vi "作业4和5 .vi"() -> ()   [LabVIEW 2018]
panel:
  in  "输入":dbl
  out "累加值":dbl
  out "等级":string
  in  "成绩":dbl
  out "是否是素数":bool
  in  "input":dbl
  out "求和":dbl
  out "布尔5":bool
  out "布尔4":bool
  out "布尔3":bool
  out "布尔2":bool
  out "布尔1":bool
  in  "间隔时间（ms）":dbl(slide) scale=0.0..1000.0
  in  "停止":bool
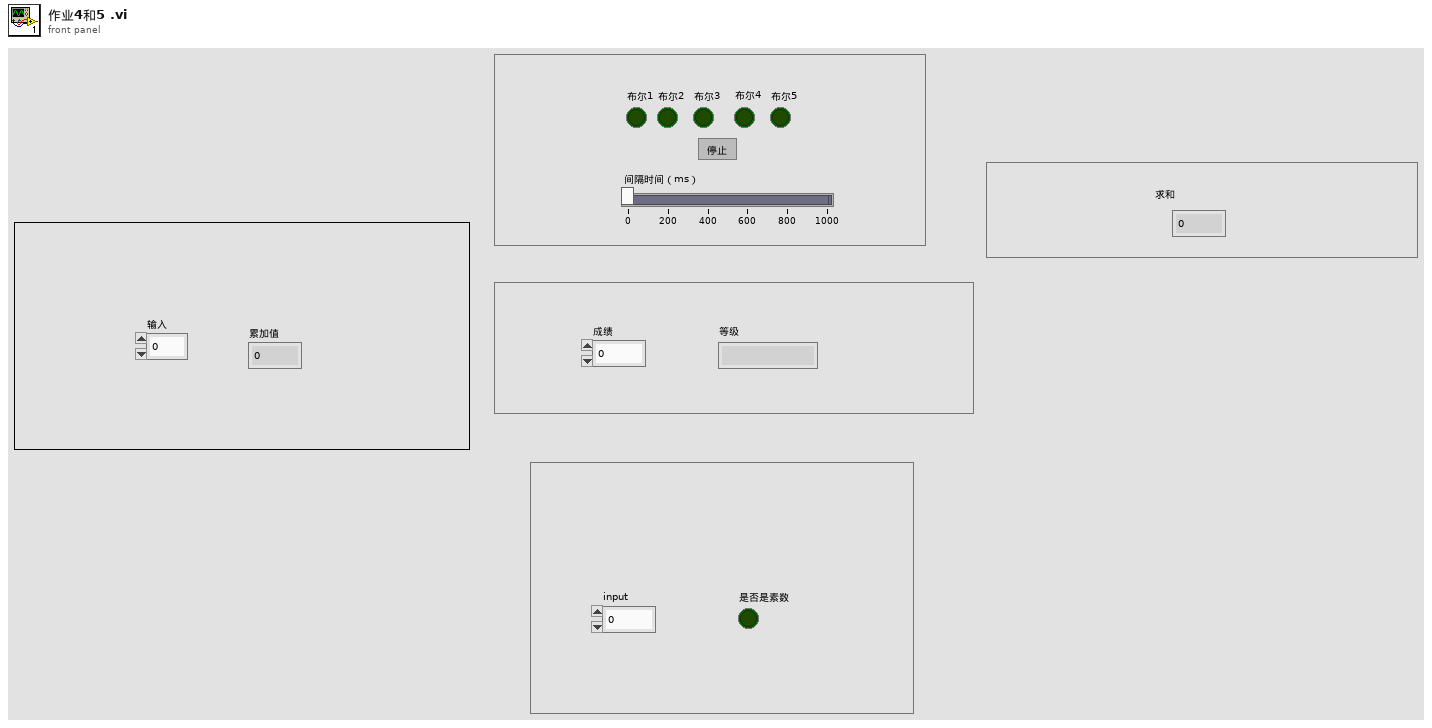
[diagram p1: front panel]
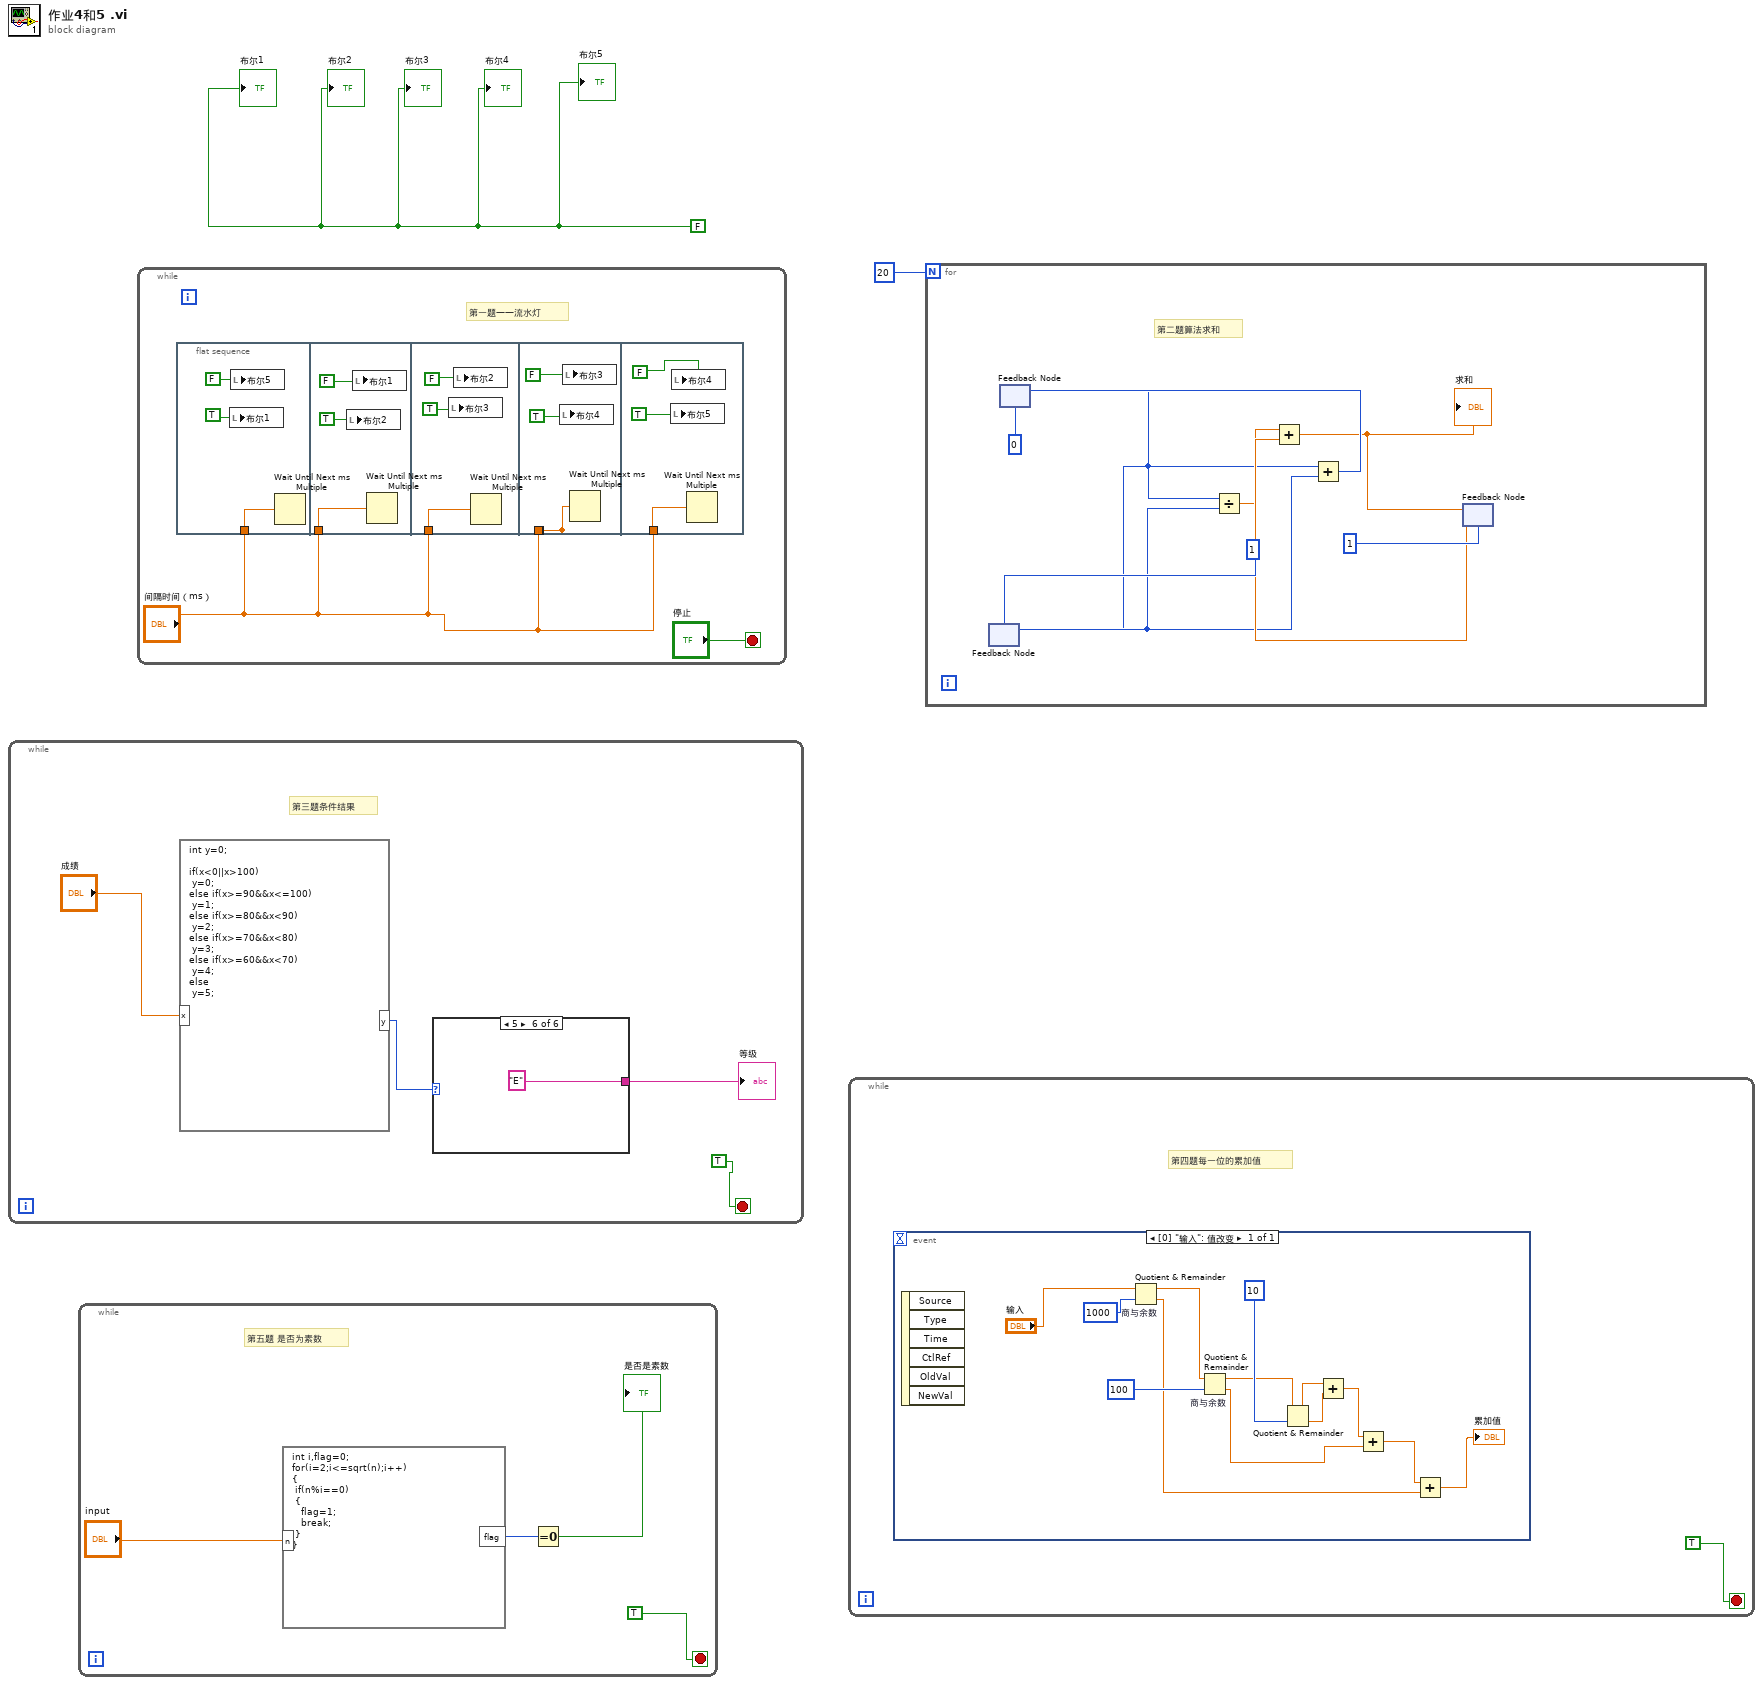
[diagram p0: block diagram]
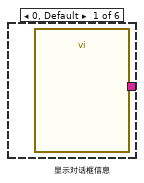
[diagram p2: hidden frame]
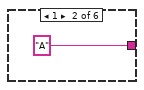
[diagram p3: hidden frame]
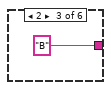
[diagram p4: hidden frame]
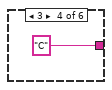
[diagram p5: hidden frame]
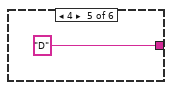
[diagram p6: hidden frame]
diagram:
  w2 = FALSE
  n1 = while {
    stop <- TRUE stop-if-true
    # "第三题条件结果"
    n2 = formula code="int y=0;\n\nif(x<0||x>100)\n y=0;\nelse if(x>=90&&x<=100)\n y=1;\nelse if(x>=80&&x<90)\n y=2;\nelse if(x>=70&&x<80)\n y=3;\nelse if(x>=60&&x<70)\n y=4;\nelse\n y=5;"("x"="成绩") -> ("y"=w4:i32)
    n3 = case shown="5" w4 {
      tunnel: [_ "A" "B" "C" "D" "E"] -> w3
      frame 0, Default {
        n4 = call "显示对话框信息"() -> ()  [unwired: 10 in, 2 out]
      }
      frame 1 {
      }
      frame 2 {
      }
      frame 3 {
      }
      frame 4 {
      }
      frame 5 {
      }
    }
    "等级" <- w3
  }
  n5 = while {
    stop <- TRUE stop-if-true
    # "第五题 是否为素数"
    n6 = formula code="int i,flag=0;\nfor(i=2;i<=sqrt(n);i++)\n{\n if(n%i==0)\n {\n   flag=1;\n   break;\n }\n}"("n"="input") -> ("flag"=w14:i32)
    n7 = Equal To 0?(x=w14) -> (x = 0?=→"是否是素数":bool)
  }
  n8 = while {
    stop <- "停止" stop-if-true
    # "第一题——流水灯"
    n9 = flat-sequence {
      tunnel: "间隔时间（ms）" -> [w18]
      tunnel: "间隔时间（ms）" -> [w21]
      tunnel: "间隔时间（ms）" -> [w24]
      tunnel: [w27] -> _
      tunnel: "间隔时间（ms）" -> [w27]
      tunnel: "间隔时间（ms）" -> [w30]
      frame #0 {
        n10 = local write "布尔1"(TRUE) -> ()
        n11 = local write "布尔5"(FALSE) -> ()
        n12 = Wait Until Next ms Multiple(millisecond multiple=w18) -> ()  [unwired: 1 out]
      }
      frame #1 {
        n13 = local write "布尔2"(TRUE) -> ()
        n14 = local write "布尔1"(FALSE) -> ()
        n15 = Wait Until Next ms Multiple(millisecond multiple=w21) -> ()  [unwired: 1 out]
      }
      frame #2 {
        n16 = local write "布尔3"(TRUE) -> ()
        n17 = local write "布尔2"(FALSE) -> ()
        n18 = Wait Until Next ms Multiple(millisecond multiple=w24) -> ()  [unwired: 1 out]
      }
      frame #3 {
        n19 = local write "布尔4"(TRUE) -> ()
        n20 = local write "布尔3"(FALSE) -> ()
        n21 = Wait Until Next ms Multiple(millisecond multiple=w27) -> ()  [unwired: 1 out]
      }
      frame #4 {
        n22 = local write "布尔5"(TRUE) -> ()
        n23 = local write "布尔4"(FALSE) -> ()
        n24 = Wait Until Next ms Multiple(millisecond multiple=w30) -> ()  [unwired: 1 out]
      }
    }
  }
  n25 = while {
    stop <- TRUE stop-if-true
    # "第四题每一位的累加值"
  }
  n26 = event shown="[0] \"输入\": 值改变" {
    selector: _ -> [_]
    dyn-events: _ -> [_]
    timeout: _ -> [_]
    event "输入": Value Change {
      n27 = event-data() -> ()  [unwired: 1 in, 6 out]
      n28 = Quotient & Remainder "商与余数"(x="输入", y=1000) -> (x-y*floor(x/y)=w37:dbl, floor(x/y)=w35:dbl)
      n29 = Quotient & Remainder "商与余数"(x=w37, y=100) -> (x-y*floor(x/y)=w43:dbl, floor(x/y)=w45:dbl)
      n30 = Quotient & Remainder(x=w43, y=10) -> (x-y*floor(x/y)=w42:dbl, floor(x/y)=w41:dbl)
      n31 = Add(x=w42, y=w41) -> (x+y=w40:dbl)
      n32 = Add(x=w40, y=w45) -> (x+y=w36:dbl)
      n33 = Add(x=w36, y=w35) -> (x+y=→"累加值":dbl)
    }
  }
  n34 = for {
    N: 20 -> [_]
    # "第二题算法求和"
    n35 = feedback #1(1) -> (w50:i32)
    n36 = feedback #2(0) -> (w48:i32)
    n37 = feedback-in #1(w48) -> ()
    n38 = Divide(x=w48, y=w50) -> (x/y=w51:dbl)
    n39 = Add(x=w48, y=w50) -> (x+y=w49:i32)
    n40 = feedback-in #2(w49) -> ()
    n41 = feedback #3 ("反馈节点")(1) -> (w52:dbl)
    n42 = Add(x=w51, y=w52) -> (x+y=w47:dbl)
    "求和" <- w47
    n43 = feedback-in #3(w47) -> ()
  }
  "布尔1" <- w2
  "布尔2" <- w2
  "布尔3" <- w2
  "布尔4" <- w2
  "布尔5" <- w2
